vi "create filepath list.vi"(2 "regular expression":string, 3 "search subholder":bool, 4 "path":path) -> (0 "num of files":i32, 1 "Array":path[](array[path]))   [LabVIEW 2018]
uses:
  <vilib>/regexp/Match Regular Expression.xnode
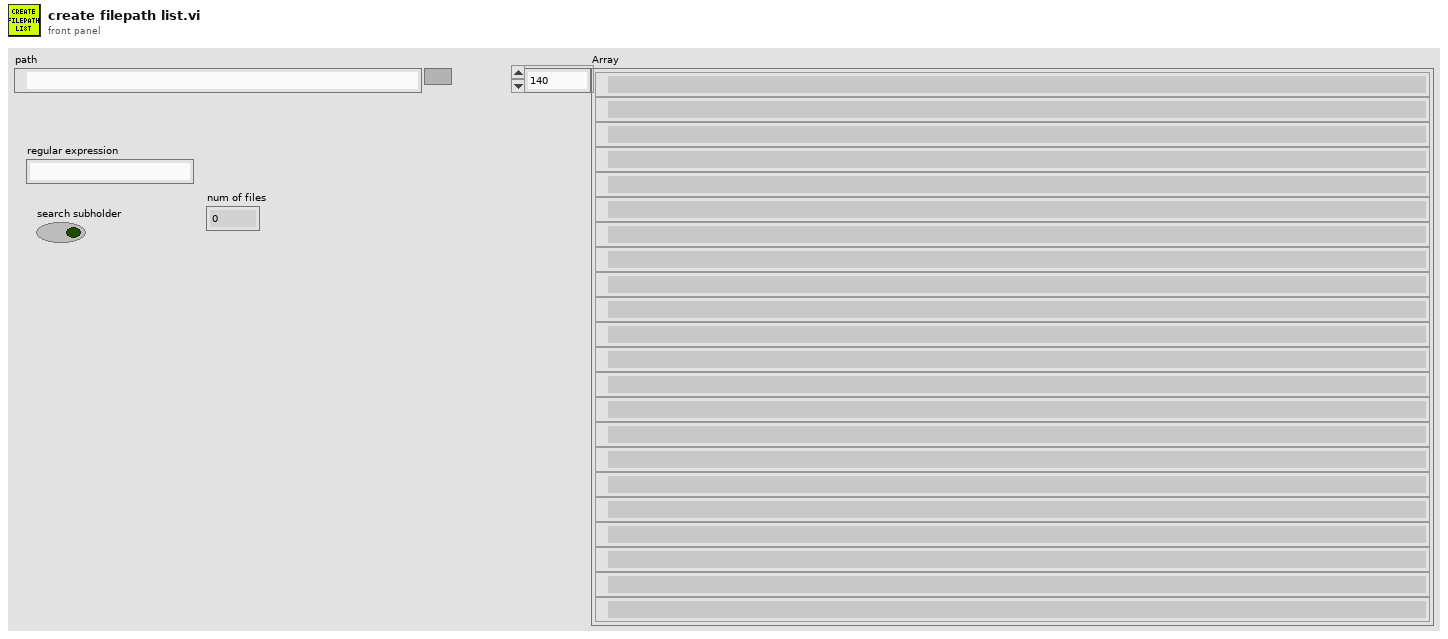
[diagram p1: front panel]
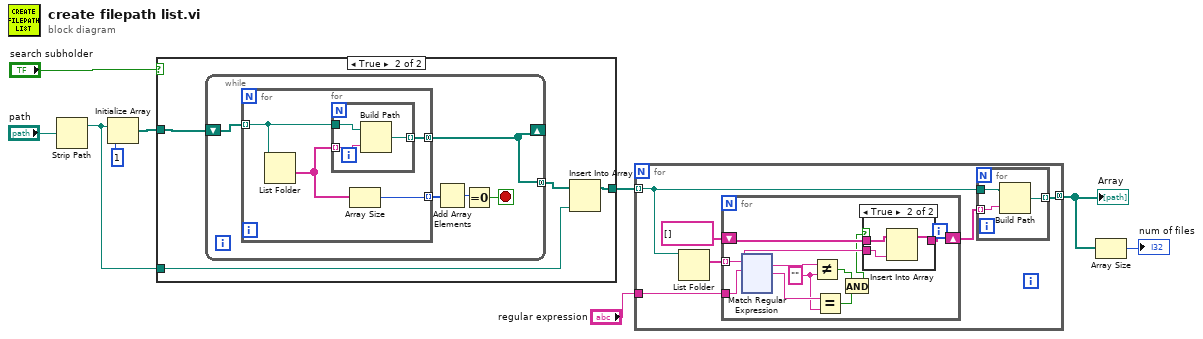
[diagram p0: block diagram]
diagram:
  n1 = Strip Path(path="path") -> (stripped path=w4:path)  [unwired: 1 out]
  n2 = Initialize Array(w4, 1 ("dimension size")) -> (w5:path[])
  n3 = case shown="True" "search subholder" {
    tunnel: w5 -> [w10 w13]
    tunnel: w4 -> [_ w12]
    tunnel: [w10 w11] -> w3
    frame False {
    }
    frame True {
      n4 = while {
        shift-right: [w15] -> _
        shift-left: w13 -> [w19]
        tunnel: [w15] -> w14 mode=concatenating
        stop <- w16 stop-if-true
        n5 = for {
          tunnel: w19 -> [w23] mode=indexing
          tunnel: [w22] -> w15 mode=concatenating
          tunnel: [w20] -> w18 mode=indexing
          n6 = List Folder(path=w23) -> (folder names=w21:string[])  [unwired: 3 in, 3 out]
          n7 = for {
            tunnel: w21 -> [w26] mode=indexing
            tunnel: w23 -> [w25]
            tunnel: [w24] -> w22 mode=indexing
            n8 = Build Path(base path=w25, name or relative path=w26) -> (appended path=w24:path)
          }
          n9 = Array Size(array=w21) -> (size(s)=w20:i32)
        }
        n10 = Add Array Elements(numeric array=w18) -> (sum=w17:i32)
        n11 = Equal To 0?(x=w17) -> (x = 0?=w16:bool)
      }
      n12 = Insert Into Array(array=w14, new element=w12) -> (w11:path[])  [unwired: 1 in]
    }
  }
  n13 = for {
    tunnel: [w32] -> w2 mode=concatenating
    tunnel: "regular expression" -> [w28]
    tunnel: w3 -> [w27] mode=indexing
    n14 = List Folder(path=w27) -> (filenames=w30:string[])  [unwired: 3 in, 3 out]
    n15 = for {
      tunnel: w30 -> [w40] mode=indexing
      shift-right: [w41] -> w29
      shift-left: string[] [] -> [w42]
      tunnel: w28 -> [w33]
      w37 = ""
      n16 = xnode "Match Regular Expression"("input string"=w40, "regular expression"=w33) -> ("whole match"=w39:string, "after match"=w38:string)  [unwired: 4 in, 3 out]
      n17 = Not Equal?(x=w39, y=w37) -> (x != y?=w36:bool)
      n18 = Equal?(x=w38, y=w37) -> (x = y?=w35:bool)
      n19 = And(x=w36, y=w35) -> (x .and. y?=w34:bool)
      n20 = case shown="True" w34 {
        tunnel: w42 -> [w43 w46]
        tunnel: [w43 w45] -> w41
        tunnel: w40 -> [_ w44]
        frame False {
        }
        frame True {
          n21 = Insert Into Array(array=w46, new element=w44) -> (w45:string[])  [unwired: 1 in]
        }
      }
    }
    n22 = for {
      tunnel: w29 -> [w163] mode=indexing
      tunnel: w27 -> [w162]
      tunnel: [w161] -> w32 mode=indexing
      n23 = Build Path(base path=w162, name or relative path=w163) -> (appended path=w161:path)
    }
  }
  "Array" <- w2
  n24 = Array Size(array=w2) -> (size(s)=→"num of files":i32)
